vi "Test Add Clears Redo.vi"(11 "Test Case In":refnum<class "Undo Redo Core.lvclass">) -> (3 "Test Case Out":refnum<class "Undo Redo Core.lvclass">)   [LabVIEW 2021, in "Undo Redo Core.lvclass"]
uses:
  Undo Redo Core.lvclass
  C:/Program Files/National Instruments/LabVIEW 2024/vi.lib/Astemes/LUnit/Test Case.lvclass
  <resource>/plugins/NIIconEditor/Controls/Undo Redo Action.ctl
  <vilib>/Astemes/LUnit/Test Case.lvclass/Test Case.ctl
  2e78792c-fd7a-40b7-88a8-0024134a4740.vi
  d374c4ae-0456-4ebf-b145-8753cc394ed2.vi
  <vilib>/Astemes/LUnit/Append Pass Result.vi
  <vilib>/Astemes/LUnit/Append Fail Result.vi
  2e78792c-fd7a-40b7-88a8-0024134a4740.vi/9c5d11cd-9439-4240-a1ee-d9baace9c924.vi
  d374c4ae-0456-4ebf-b145-8753cc394ed2.vi/9c5d11cd-9439-4240-a1ee-d9baace9c924.vi
  <vilib>/Astemes/LUnit/Run In UI.vi
  <vilib>/Utility/error.llb/Clear Errors.vi
  <vilib>/Astemes/LUnit/Test Case.lvclass
panel:
  out "State After Redo":string
  out "error out":errorcluster
  out "State After Adding":string
  out "Undo State Outputs":string[](array[string])
  out "State After Initial Adding":string
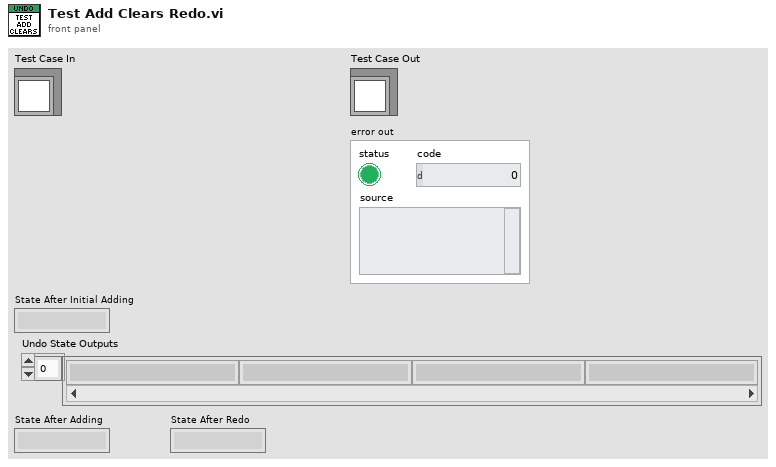
[diagram p1: front panel]
types:
  T1 = typedef "Undo Redo Action.ctl" = enum16{"Init", "Add", "Undo", "Redo", "Current State"}
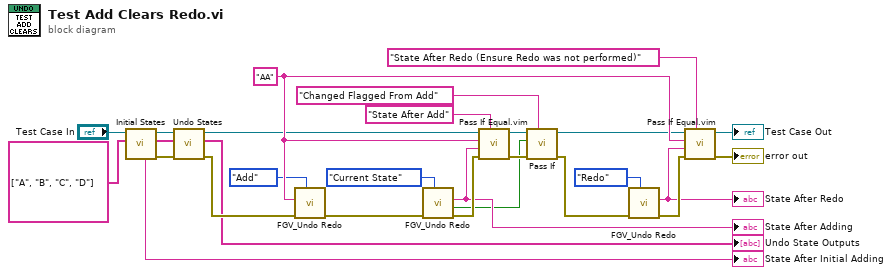
[diagram p0: block diagram]
diagram:
  w20 = "AA" ("Data in")
  n1 = call "Initial States.vi"("States"=string[] ["A", "B", "C", "D"], "Test Case In"="Test Case In") -> ("error out"=w26:errorcluster, "Expected Undo Stack"=w10:string[], "Test Case Out"=w13:refnum<class "Undo Redo Core.lvclass">, "Current State"=→"State After Initial Adding":string)  [unwired: 6 in]
  n2 = call "Undo States.vi"("error in"=w26, "Expected Undo States"=w10, "Test Case In"=w13) -> ("error out"=w25:errorcluster, "Actual Undo States"=→"Undo State Outputs":string[], "Test Case Out"=w17:refnum<class "Undo Redo Core.lvclass">)  [unwired: 5 in, 1 out]
  n3 = call <resource>:"FGV_Undo Redo.vi"("Action"=Undo_Redo_Action."Add", "error in"=w25, "State In"=w20) -> ("error out"=w27:errorcluster)  [unwired: 6 in, 2 out]
  n4 = call <resource>:"FGV_Undo Redo.vi"("Action"=Undo_Redo_Action."Current State", "error in"=w27) -> ("error out"=w28:errorcluster, "Have Changes"=w1:bool, "State Out"=w6:string)  [unwired: 7 in]
  "State After Adding" <- w6
  n5 = call "Pass If Equal.vim"("Description"="State After Add", "error in (no error)"=w28, "Actual"=w6, "Expected"=w20, "LUnit Test Case In"=w17) -> ("error out"=w22:errorcluster, "LUnit Test Case Out"=w4:refnum<class "Undo Redo Core.lvclass">)  [unwired: 5 in]
  n6 = call <vilib>:"Pass If.vi"("Description"="Changed Flagged From Add", "error in (no error)"=w22, "Pass?"=w1, "LUnit Test Case In"=w4) -> ("error out"=w21:errorcluster, "LUnit Test Case Out"=w3:refnum<class "Undo Redo Core.lvclass">)  [unwired: 6 in]
  n7 = call <resource>:"FGV_Undo Redo.vi"("Action"=Undo_Redo_Action."Redo", "error in"=w21) -> ("error out"=w23:errorcluster, "State Out"=w5:string)  [unwired: 7 in, 1 out]
  "State After Redo" <- w5
  n8 = call "Pass If Equal.vim"("Description"="State After Redo (Ensure Redo was not performed)", "error in (no error)"=w23, "Actual"=w5, "Expected"=w20, "LUnit Test Case In"=w3) -> ("error out"=→"error out":errorcluster, "LUnit Test Case Out"=→"Test Case Out":refnum<class "Undo Redo Core.lvclass">)  [unwired: 5 in]
